vi "play-simple-force-mapping.vi"() -> ()   [LabVIEW 2017]
uses:
  <vilib>/userdefined/High Color/nirio_resource_hc.ctl
  <vilib>/FPGAPlugInAG/cRIO-9082/niLvFpga_Open_cRIO-9082.vi
  <vilib>/rvi/interface/common/dynamic/niFpgaDynamicAddResources.vi
  <vilib>/FPGAPlugInAG/Dynamic/niLvFpga_Reset_Dynamic.vi
  <vilib>/rvi/interface/common/niFpgaWaitOnOcc.vi
  <vilib>/Utility/error.llb/Error Cluster From Error Code.vi
  <vilib>/rvi/errors/niLvFpgaAdjustHostInterfaceError.vi
  <vilib>/FPGAPlugInAG/Dynamic/niLvFpga_Run_Dynamic.vi
  <vilib>/Utility/file.llb/Write Delimited Spreadsheet (DBL).vi
  <vilib>/FPGAPlugInAG/Dynamic/niLvFpga_Close_Dynamic.vi
  <vilib>/rvi/interface/nirviOpenFPGA/nirviOpenFPGA.xnode
  FPGA Bitfiles/afmimagingcontro_FPGATargetSPARTA_simple-force-map_FwCwu-swAI0.lvbitx
  <vilib>/rvi/interface/nirviMethod/nirviMethod.xnode
  <vilib>/rvi/interface/nirviReadWriteControl/nirviReadWriteControl.xnode
  <vilib>/rvi/interface/nirviCloseFPGA/nirviCloseFPGA.xnode
  <vilib>/FPGAPlugInAG/Dynamic/niLvFpga_ConfigureFifo_Dynamic.vi
  <vilib>/rvi/errors/niLvFpgaMergeErrorWithErrorCode.vi
  <vilib>/rvi/interface/Simulation/niFpgaSimulationCallBeginRW.vi
  <vilib>/FPGAPlugInAG/Dynamic/niLvFpga_ReadFifo_Dynamic.vi
  NiFpgaLv.dll
  controls/expMetaData.ctl
  <userlib>/_matio/level5.lvlib
  <userlib>/_matio/level5/Public/Write/Append Data Element.llb/Append Data Element (Anything).vi
panel:
  out "Current Case 2":i16
  out "Numeric":i32
  in  "sysID_Z_axis_params":T1={"TOL"=0.3, "ramp-rate"=-5e-05, "z-u-max"=0.0, "offset"=0.0, "Ki"=0.005, "Z-error-threshold"=0.05, "Z-settled-samples\nthreshold "=0, "z_UP"=0.0, "zup-N"=0}
  out "result string":string
  out "boolean  indicators":T2
  in  "Tab Control":enum32{"Main Settings", "Host Debug"}(tab)
  in  "init Z up":sgl step=0.5
  in  "trigger-0":bool
  in  "outputData":path=path "C:/Users/arnold/Documents/labview/afm_imaging/data/data-out.csv"
  in  "TsTicks":u32=1600
  out "e(0) (threshhold init)":fxp<+/-,16,5>
  in  "z-down-max":fxp<+/-,32,16>
  out "Current Case":i16
  out "iter":i32
  out "size(s)":i32
  out "y iter":i32
  out "size(s) 2":i32[](array[numeric])
  out "Array":i32[][](array[numeric])
  out "z-control":dbl[](graph)
  out "z-error":dbl[](graph)
  in  "STOP":bool
  # "- If collect all = fasle and collect move = false,\nwe only collect measurement data.\n- If collect all = false, and collect move = true,\nwe collect measurement and move data.\n- If collect all = true, we collect everything."
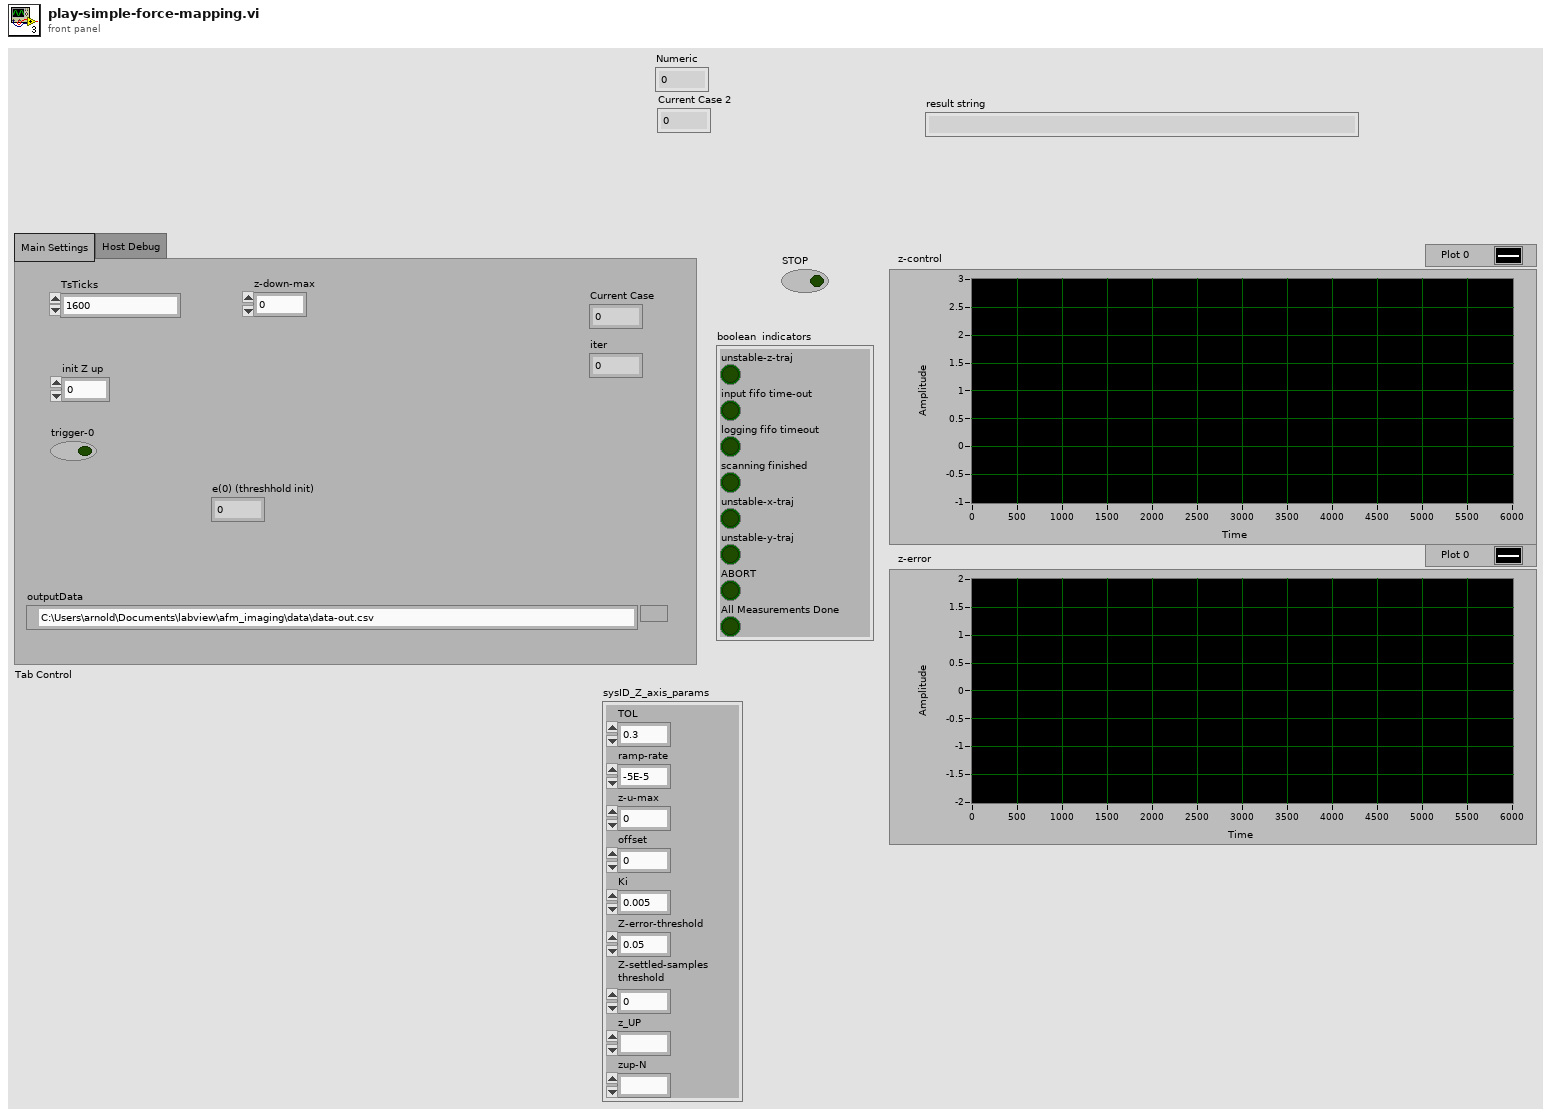
[diagram p1: front panel]
types:
  T1 = cluster{"TOL":sgl, "ramp-rate":sgl, "z-u-max":sgl, "offset":sgl, "Ki":sgl, "Z-error-threshold":sgl, "Z-settled-samples\nthreshold ":i16, "z_UP":fxp<+/-,16,5>, "zup-N":i16}
  T2 = cluster{"unstable-z-traj":bool, "input fifo time-out":bool, "logging fifo timeout":bool, "scanning finished":bool, "unstable-x-traj":bool, "unstable-y-traj":bool, "ABORT":bool, "All Measurements Done":bool}
  T3 = typedef "nirio_resource_hc.ctl" = tag
  T4 = enum16{"open", "replace", "create", "open or create", "replace or create", "replace or create with confirmation"}
  T5 = typedef "expMetaData.ctl" = cluster{"xy_error_threshold":sgl, "xy_settled_samples_threshold":i16, "Ki_xy":sgl, "state_counts":dbl[], "TOL":sgl, "ramp_rate":sgl, "z_u_max":sgl, "setpoint":sgl, "Ki":sgl, "Z_error_threshold":sgl, "Z_settled_samples_threshold ":i16, "z_UP":sgl, "zup_N":i16, "Num":sgl[], "Den":sgl[], "max_Z_settle_samples":i16, "Kiz_down":sgl, "do_xy_CL":bool, "do_Alt_Ztrigger":bool, "output-data-path":path, "input-data-path":path}
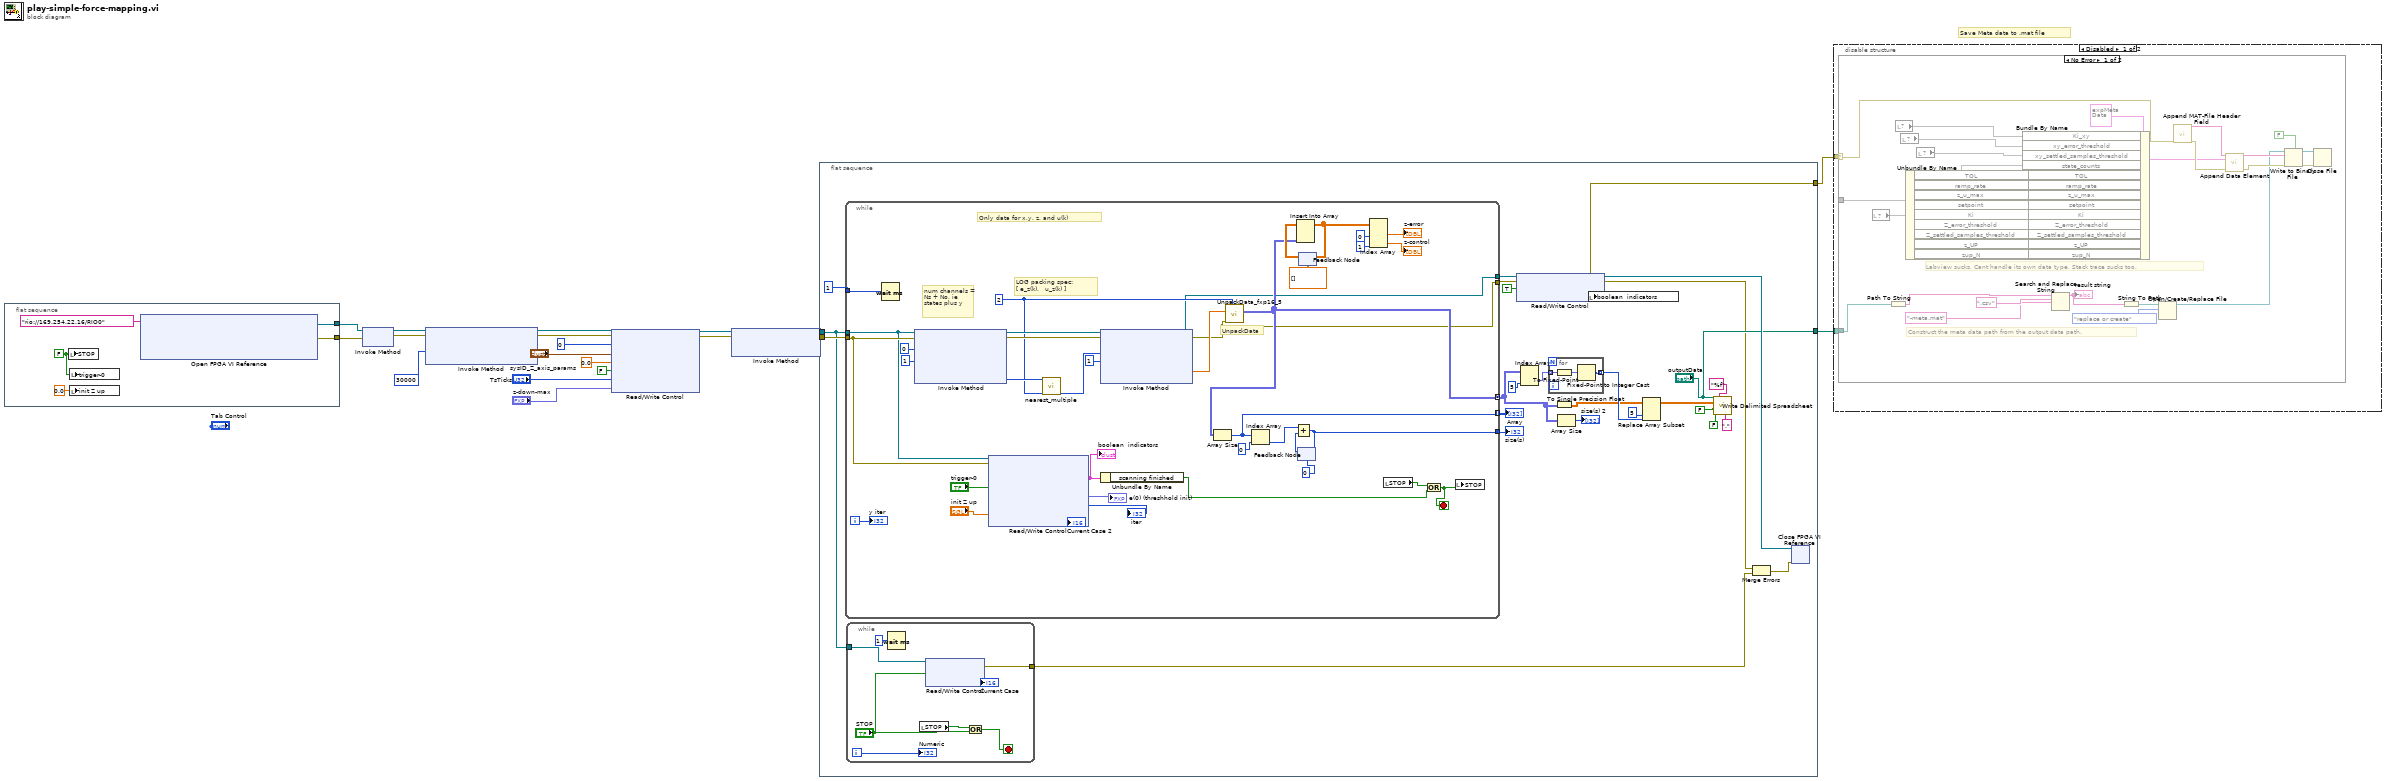
[diagram p0: block diagram]
diagram:
  # "Save Meta data to .mat file"
  n1 = flat-sequence {
    tunnel: [w24] -> w18
    tunnel: [w23] -> w17
    frame #0 {
      w21 = FALSE ("STOP")
      n2 = local write "STOP"(w21) -> ()
      n3 = local write "trigger-0"(w21) -> ()
      n4 = local write "init Z up"(sgl 0.0 ("init Z up")) -> ()
      n5 = xnode "Open FPGA VI Reference"("resource name"=T3 "rio://169.254.22.16/RIO0") -> ("FPGA VI Reference Out"=w24:refnum<k20>, "error out"=w23:errorcluster)  [unwired: 1 in]
    }
  }
  n6 = xnode "Invoke Method"("FPGA VI Reference In"=w18, "error in"=w17) -> ("FPGA VI Reference Out"=w16:refnum<k20>, "error out"=w15:errorcluster)
  n7 = xnode "Invoke Method"("FPGA VI Reference In"=w16, "error in"=w15, "Requested Depth"=30000) -> ("FPGA VI Reference Out"=w6:refnum<k20>, "error out"=w5:errorcluster)  [unwired: 1 out]
  n8 = xnode "Read/Write Control"("FPGA VI Reference In"=w6, "error in"=w5, "initial case"=i16 0, "sysID_Z_axis_params"="sysID_Z_axis_params", "init Z up"=sgl 0.0 ("u(0)"), "trigger-0"=FALSE, "TsTicks"="TsTicks", "z-down-max"="z-down-max") -> ("FPGA VI Reference Out"=w2:refnum<k20>, "error out"=w1:errorcluster)
  n9 = xnode "Invoke Method"("FPGA VI Reference In"=w2, "error in"=w1) -> ("FPGA VI Reference Out"=w4:refnum<k20>, "error out"=w3:errorcluster)  [unwired: 1 in]
  n10 = flat-sequence {
    tunnel: w3 -> [w48]
    tunnel: w4 -> [w38]
    tunnel: [w25] -> w9
    tunnel: ["outputData"] -> w10
    frame #0 {
      n11 = while {
        tunnel: 1 -> [w99]
        tunnel: w38 -> [w88]
        tunnel: w48 -> [w89]
        tunnel: [w66] -> w43
        tunnel: [w71] -> w30 mode=concatenating
        tunnel: [w86] -> w49
        tunnel: [w69] -> w42
        tunnel: [w78] -> w37 mode=indexing
        i -> [w87]
        stop <- w79 stop-if-true
        w72 = u32 2 ("y")
        # "LOG packing spec:\n[ e_z(k),   u_z(k) ]"
        # "num channels = Ns + No, ie states plus y"
        # "Only data for x,y, z, and u(k)"
        # "UnpackData"
        n12 = Wait (ms)(milliseconds to wait=w99) -> ()  [unwired: 1 out]
        n13 = xnode "Invoke Method"("FPGA VI Reference In"=w88, "error in"=w89, "Number of Elements"=0 ("Timeout (ms)"), "Timeout (ms)"=1) -> ("FPGA VI Reference Out"=w95:refnum<k20>, "error out"=w96:errorcluster, "Elements Remaining"=w83:u32)  [unwired: 1 out]
        n14 = xnode "Read/Write Control"("FPGA VI Reference In"=w88, "error in"=w89, "trigger-0"="trigger-0", "init Z up"="init Z up") -> ("boolean  indicators"=w81:T2, "e(0) (threshhold init)"=→"e(0) (threshhold init)":fxp<+/-,16,5>, "iter"=→"iter":i32, "Current Case"=→"Current Case 2":i16)  [unwired: 1 in, 2 out]
        "boolean  indicators" <- w81
        n15 = call "nearest_multiple.vi"("numChan"=w72, "N"=w83) -> ("(int) y*floor(x/y)"=w82:u64)  [unwired: 9 in]
        n16 = xnode "Invoke Method"("FPGA VI Reference In"=w95, "error in"=w96, "Number of Elements"=w82, "Timeout (ms)"=1) -> ("FPGA VI Reference Out"=w66:refnum<k20>, "error out"=w69:errorcluster, "Data"=w70:sgl[])  [unwired: 1 out]
        n17 = Unbundle By Name(w81) -> ("scanning finished"=w68:bool)
        n18 = call "UnpackData_fxp16_5.vi"("NumChannels"=w72, "error In"=w69, "1D Data In"=w70) -> ("2D Data Out"=w71:fxp<+/-,16,5>[][])  [unwired: 7 in, 1 out]
        n19 = Array Size(array=w71) -> (size(s)=w78:i32[])
        n20 = Index Array(array=w78, index=0) -> (element=w91:i32)
        n21 = feedback #1(0) -> (w92:i32)
        n22 = Add(x=w91, y=w92) -> (x+y=w86:i32)
        n23 = feedback-in #1(w86) -> ()
        n24 = feedback #2(dbl[][] []) -> (w76:dbl[][])
        n25 = Insert Into Array(array=w76, new element=w71) -> (w73:dbl[][])  [unwired: 2 in]
        n26 = feedback-in #2(w73) -> ()
        n27 = Index Array(array=w73, index (col) #1=0 ("disabled index (col)"), index (col) #2=1 ("index (col)")) -> (element #1=→"z-error":dbl[], element #2=→"z-control":dbl[])  [unwired: 2 in]
        n28 = local read "STOP"() -> (w80:bool)
        n29 = Or(x=w80, y=w68) -> (x .or. y?=w79:bool)
        n30 = local write "STOP"(w79) -> ()
        "y iter" <- w87
      }
      "size(s)" <- w49
      "Array" <- w37
      n31 = while {
        tunnel: w38 -> [w61]
        tunnel: [w54] -> w27
        i -> [w55]
        stop <- w57 stop-if-true
        n32 = Wait (ms)(milliseconds to wait=u32 1) -> ()  [unwired: 1 out]
        n33 = local read "STOP"() -> (w58:bool)
        n34 = xnode "Read/Write Control"("FPGA VI Reference In"=w61, "ABORT"="STOP") -> ("error out"=w54:errorcluster, "Current Case"=→"Current Case":i16)  [unwired: 1 in, 1 out]
        n35 = Or(x=w58, y="STOP") -> (x .or. y?=w57:bool)
        "Numeric" <- w55
      }
      n36 = xnode "Read/Write Control"("FPGA VI Reference In"=w43, "error in"=w42, "ABORT"=TRUE) -> ("FPGA VI Reference Out"=w40:refnum<k20>, "error out"=w25:errorcluster, "boolean  indicators"=w36:T2)
      n37 = Index Array(array=w30, index (col)=5) -> (element=w34:fxp<+/-,16,5>[])  [unwired: 1 in]
      n38 = for {
        tunnel: w34 -> [w52] mode=indexing
        tunnel: [w53] -> w32 mode=indexing
        n39 = To Fixed-Point(number=w52) -> (fixed-point=w51:fxp<+/-,16,5>)  [unwired: 1 in]
        n40 = Fixed-Point to Integer Cast(1:w51) -> (0:w53:i16)
      }
      n41 = To Single Precision Float(number=w30) -> (single precision float=w29:sgl[][])
      n42 = Array Size(array=w30) -> (size(s)=→"size(s) 2":i32[])
      n43 = local write "boolean  indicators"(w36) -> ()
      n44 = Replace Array Subset(array=w29, new element=w32, index (col)=5) -> (w31:sgl[][])  [unwired: 1 in]
      n45 = call-poly <vilib>:"Write Delimited Spreadsheet.vi"("file path (dialog if empty)"="outputData", "format (%.3f)"="%f", "2D data"=w31, "append to file? (new file:F)"=FALSE, "transpose? (no:F)"=FALSE, "delimiter (\\t)"=",") -> ()  [unwired: 8 in, 2 out]
      n46 = Merge Errors(w25, w27) -> (w26:errorcluster)
      n47 = xnode "Close FPGA VI Reference"("FPGA VI Reference In"=w40, "error in"=w26) -> ()  [unwired: 1 out]
    }
  }
  n48 = disable-structure shown="Disabled" {
    disable-tunnel: w10 -> [w101 _]
    disable-tunnel: w9 -> [w100 _]
    frame Disabled {
      n49 = case shown="No Error" w100 {
        selector: w100 -> [w122 _]
        tunnel: w101 -> [w103 _]
        tunnel: _ -> [w108 _]
        frame No Error {
          # "Construct the meta data path from the output data path."
          # "Labview sucks. Cant handle its own data type. Stack trace sucks too."
          n50 = local read item#-1() -> (w107)
          n51 = Path To String(path=w103) -> (string=w125:string)
          n52 = local read item#-1() -> (w106)
          n53 = local read item#-1() -> (w105)
          n54 = Unbundle By Name(w107) -> ("TOL"=w118, "ramp_rate"=w117, "z_u_max"=w116, "setpoint"=w115, "Ki"=w114, "Z_error_threshold"=w113, "Z_settled_samples_threshold"=w112, "z_UP"=w111, "zup_N"=w110)
          n55 = local read item#-1() -> (w104)
          n56 = Bundle By Name(cluster=T5 {"xy_error_threshold"=0.1, "xy_settled_samples_threshold"=200, "Ki_xy"=0.005, "state_counts"=[], "TOL"=0.3, "ramp_rate"=-5e-06, "z_u_max"=5.0, "setpoint"=0.0, "Ki"=0.001, "Z_error_threshold"=0.0, "Z_settled_samples_threshold "=0, "z_UP"=1.5, "zup_N"=5000, "Num"=[-0.00254, 0.000408, 0.00295, 0.0, 0.0, 0.0, 0.0, 0.0, 0.0], "Den"=[0.982758, -1.98194, 1.0, 0.0, 0.0, 0.0, 0.0, 0.0, 0.0], "max_Z_settle_samples"=5000, "Kiz_down"=0.001, "do_xy_CL"=FALSE, "do_Alt_Ztrigger"=FALSE, "output-data-path"=path "", "input-data-path"=path ""} ("ExpMetaData"), "Ki_xy"=w106, "xy_error_threshold"=w105, "xy_settled_samples_threshold"=w104, "state_counts"=w108, "TOL"=w118, "ramp_rate"=w117, "z_u_max"=w116, "setpoint"=w115, "Ki"=w114, "Z_error_threshold"=w113, "Z_settled_samples_threshold"=w112, "z_UP"=w111, "zup_N"=w110) -> (w119:T5)
          n57 = Search and Replace String(input string=w125, search string=".csv", replace string="-meta.mat" ("replace string (\"\")")) -> (result string=w124:string)  [unwired: 5 in, 3 out]
          "result string" <- w124
          n58 = String To Path(string=w124) -> (path=w121:path)
          n59 = Open/Create/Replace File(file path (use dialog)=w121, operation (0:open)=T4."replace or create") -> (refnum out=w120:refnum<file>)  [unwired: 4 in, 2 out]
          n60 = call <userlib>:"Append MAT-File Header Field.vi"("error"=w122) -> ("result string"=w133:string, "error out"=w123:errorcluster)  [unwired: 13 in]
          n61 = call-poly <userlib>:"Append Data Element.vi"("initial string"=w133, "data"=w119, "error in (no error)"=w123) -> ("result string"=w131:string, "error out"=w132:errorcluster)  [unwired: 11 in]
          n62 = Write to Binary File(file (use dialog)=w120, data=w131, error in=w132, 5:FALSE ("prepend array or string size? (T)")) -> (refnum out=w128:refnum<file>, error out=w129:errorcluster)  [unwired: 2 in, 1 out]
          n63 = Close File(refnum=w128, error in=w129) -> ()  [unwired: 2 out]
        }
        frame Error {
        }
      }
    }
    frame Enabled {
    }
  }
